vi "showDialog.vi"(0 "HB_OneButtonDialog in":refnum<class "HB_OneButtonDialog.lvclass">, 11 "error in (no error)":errorcluster) -> (4 "HB_OneButtonDialog out":refnum<class "HB_OneButtonDialog.lvclass">, 8 "Button Index":i16, 15 "error out":errorcluster)   [LabVIEW 2009, in "HB_Inherance_Example.lvlib" / "HB_OneButtonDialog.lvclass"]
doc: "Override VI. This VI implements the display of a one button dialog."
uses:
  HB_OneButtonDialog.lvclass
  HB_Dialog/HB_Dialog.lvclass
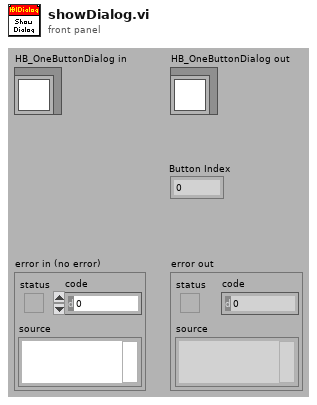
[diagram p1: front panel]
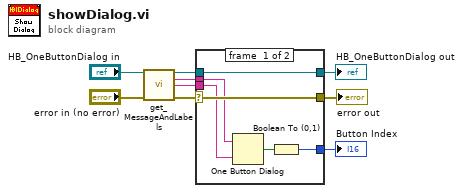
[diagram p0: block diagram]
diagram:
  n1 = call "get_MessageAndLabels.vi"("HB_Dialog in"="HB_OneButtonDialog in", "error in (no error)"="error in (no error)") -> ("HB_Dialog out"=w1:refnum<class "HB_OneButtonDialog.lvclass">, "Message"=w7:string, "T button name"=w6:string, "error out"=w4:errorcluster)  [unwired: 9 in, 1 out]
  n2 = case shown="No Error" w4 {
    selector: w4 -> [w14 w16]
    tunnel: w7 -> [w12 _]
    tunnel: w6 -> [w11 _]
    tunnel: [w10 _] -> w5
    tunnel: [w14 w16] -> w3
    tunnel: [w13 w17] -> w2
    tunnel: w1 -> [w13 w17]
    frame #0 {
      n3 = One Button Dialog(message=w12, button name ("OK")=w11) -> (true=w15:bool)
      n4 = Boolean To (0,1)(Boolean=w15) -> (0, 1=w10:i16)
    }
    frame #1 {
    }
  }
  "error out" <- w3
  "HB_OneButtonDialog out" <- w2
  "Button Index" <- w5
